vi "Get AP Sx Parameter.vi"(8 "error in (no error)":errorcluster caption="错误输入（无错误）", 9 "value":u32, 10 "asicBitsName":i32, 11 "asicHandle":i32) -> (0 "error out":errorcluster caption="错误输出", 1 "value out":u32, 3 "function return":i32)   [LabVIEW 2018]
doc: "extern int __stdcall GetAPSxParameter (int asicHandle, int asicBitsName, OUT void * value);"
uses:
  APSx.dll/APSx.dll
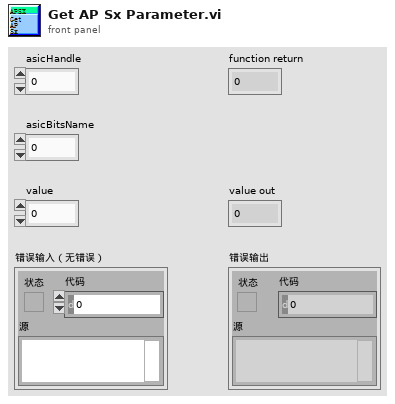
[diagram p1: front panel]
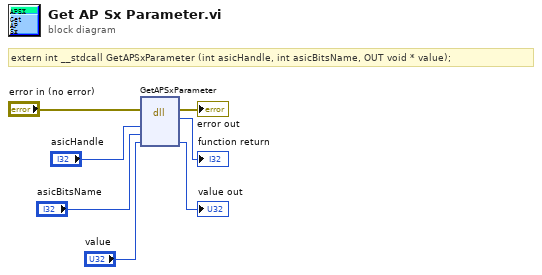
[diagram p0: block diagram]
diagram:
  # "extern int __stdcall GetAPSxParameter (int asicHandle, int asicBitsName, OUT void * value);"
  n1 = dll-call lib="PTH2[abs D项目Feng恒隆项目Labview传感器对中台SourcesAPSx.dllAPSx.*" fn="GetAPSxParameter"(error in="error in (no error)", "asicHandle"="asicHandle", "asicBitsName"="asicBitsName", "value"="value") -> (error out=→"error out":errorcluster, →"function return":i32, "value"=→"value out":u32)  [unwired: 4 in, 1 out]
